vi "exitApp.vi"(8 "error in (no error)":errorcluster, 11 "pdbm_testsys_reqst_event":refnum<user-event>) -> (0 "error IO":errorcluster, 3 "pdbm_testsys_reqst_event out":refnum<user-event>)   [LabVIEW 2015, in "pdbm_test_system.lvlib"]
uses:
  pdbm_test_system.lvlib
  pdbm_testsys_taskroute_inter/UsrDefine/pdbm_testsys_reqst_data.ctl
  pdbm_testsys_taskroute_inter/pdbm_testsys_taskroute_inter.lvlib
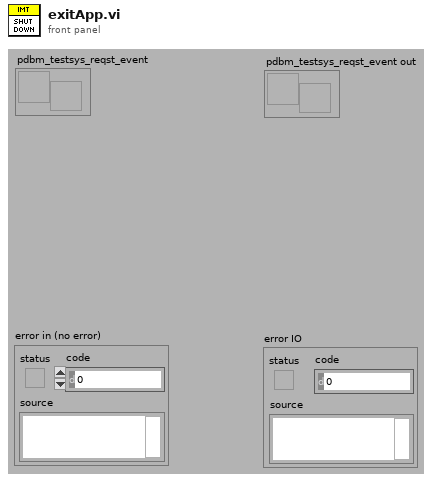
[diagram p1: front panel]
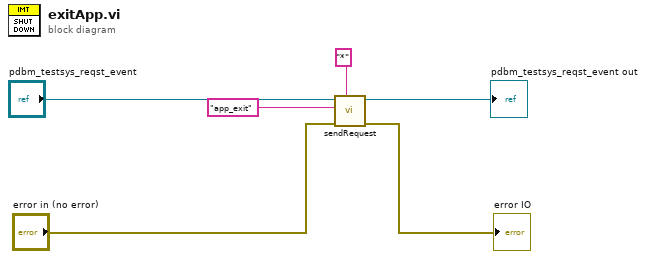
[diagram p0: block diagram]
diagram:
  n1 = call "sendRequest.vi"("TaskName"="*", "error in (no error)"="error in (no error)", "Request"="app_exit", "pdbm_testsys_reqst_event"="pdbm_testsys_reqst_event") -> ("error IO"=→"error IO":errorcluster, "pdbm_testsys_reqst_event out"=→"pdbm_testsys_reqst_event out":refnum<user-event>)  [unwired: 6 in]
